vi "Insert Into SubPanel.vi"(8 "error in (no error)":errorcluster, 10 "SubPanel Ref":refnum<vi>, 11 "ViewableActor in":refnum<class "ViewableActor.lvclass">) -> (0 "error out":errorcluster, 3 "ViewableActor out":refnum<class "ViewableActor.lvclass">)   [LabVIEW 2020, in "ViewableActor.lvlib" / "ViewableActor.lvclass"]
uses:
  ViewableActor.lvclass
  ViewableActor.lvclass/ViewableActor.ctl
  Write SubPanel Ref.vi
  Read SubPanel Ref.vi
  Read UI VI Ref.vi
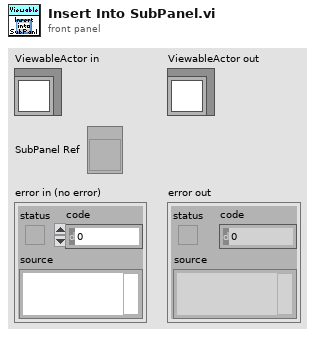
[diagram p1: front panel]
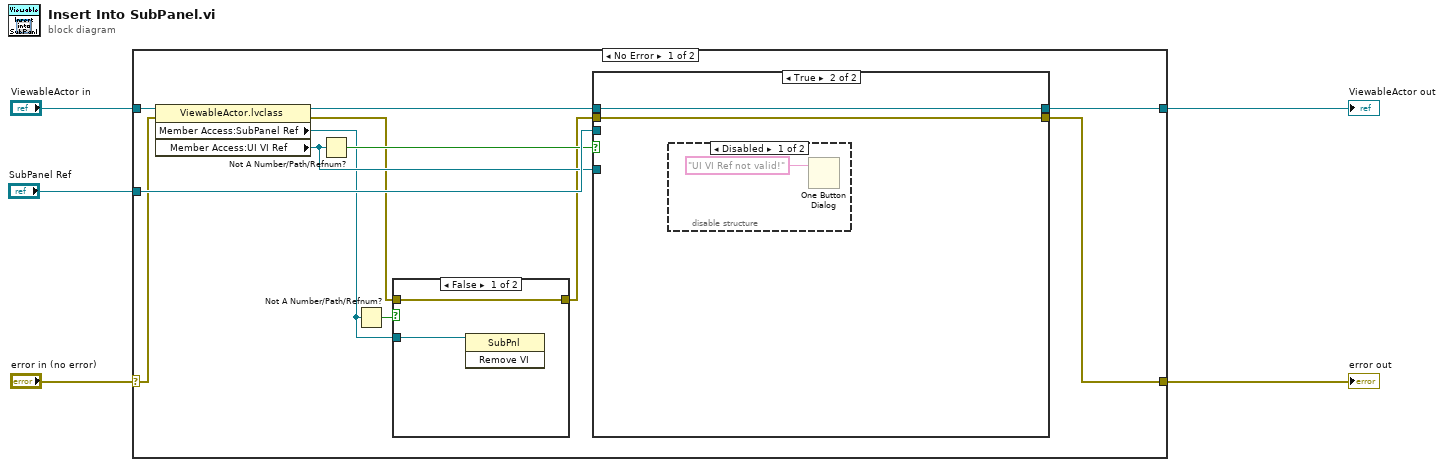
[diagram p0: block diagram]
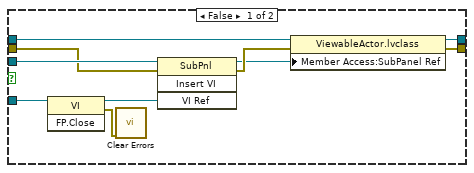
[diagram p3: hidden frame]
diagram:
  n1 = case shown="No Error" "error in (no error)" {
    selector: "error in (no error)" -> [w11 w35]
    tunnel: [w6 w35] -> w4
    tunnel: [w15 w34] -> w2
    tunnel: "ViewableActor in" -> [w17 w34]
    tunnel: "SubPanel Ref" -> [w14 _]
    frame No Error {
      n2 = property class="ViewableActor.lvclass"(reference=w17, error in=w11) -> (reference out=w16:refnum<class "ViewableActor.lvclass">, error out=w8:errorcluster, "Member Access:SubPanel Ref"=w9:refnum<vi>, "Member Access:UI VI Ref"=w12:refnum<vi>)
      n3 = Not A Number/Path/Refnum?(number/path/refnum=w12) -> (NaN/Path/Refnum?=w13:bool)
      n4 = Not A Number/Path/Refnum?(number/path/refnum=w9) -> (NaN/Path/Refnum?=w10:bool)
      n5 = case shown="False" w10 {
        tunnel: w9 -> [w19 _]
        tunnel: w8 -> [w18 w20]
        tunnel: [w18 w20] -> w7
        frame False {
          n6 = invoke on="Invoke Node" class="SubPnl" method="Remove VI"(reference=w19) -> ()  [unwired: 2 in, 3 out]
        }
        frame True {
        }
      }
      n7 = case shown="True" w13 {
        tunnel: w16 -> [w29 w32]
        tunnel: [w28 w32] -> w15
        tunnel: w14 -> [w27 _]
        tunnel: w12 -> [w22 _]
        tunnel: w7 -> [w25 w31]
        tunnel: [w24 w31] -> w6
        frame False {
          n8 = invoke class="VI" method="FP.Close"(reference=w22) -> (reference out=w30:refnum<vi>, error out=w21:errorcluster)  [unwired: 2 in, 1 out]
          n9 = call <vilib>:"Clear Errors.vi"("error in (no error)"=w21) -> ()  [unwired: 5 in, 2 out]
          n10 = invoke on="Invoke Node" class="SubPnl" method="Insert VI"(reference=w27, error in=w25, "VI Ref"=w30) -> (reference out=w23:refnum<vi>, error out=w26:errorcluster)  [unwired: 1 in, 2 out]
          n11 = property class="ViewableActor.lvclass"(reference=w29, error in=w26, "Member Access:SubPanel Ref"=w23) -> (reference out=w28:refnum<class "ViewableActor.lvclass">, error out=w24:errorcluster)
        }
        frame True {
          n12 = disable-structure shown="Disabled" {
            frame Disabled {
              n13 = One Button Dialog(message="UI VI Ref not valid!") -> ()  [unwired: 1 in, 1 out]
            }
            frame Enabled {
            }
          }
        }
      }
    }
    frame Error {
    }
  }
  "error out" <- w4
  "ViewableActor out" <- w2
